vi "poly_recursive_compare_cluster_element(s).vi"(6 "stop after 1st one?":bool, 7 "delimiter (/)":string="/", 8 "error in (no error)":errorcluster, 10 "Data":variant, 11 "Cluster":variant) -> (0 "error out":errorcluster, 1 "field names":string[](array[string]), 2 "found?":bool, 3 "Cluster out":variant)   [LabVIEW 2015]
uses:
  <vilib>/Utility/Data Type/NI_Data Type.lvlib
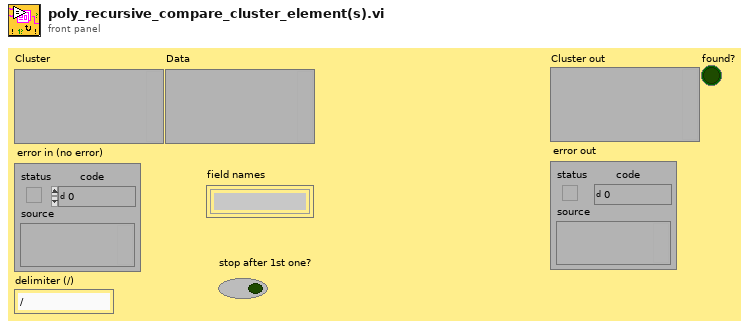
[diagram p1: front panel]
types:
  T1 = typedef "NI_Data Type.lvlib/Data Type.ctl" = enum8{"Invalid Type", "Void", "I8", "I16", "I32", "I64", "U8", "U16", "U32", "U64", "Single Float", "Double Float", "Extended Float", "Single Complex", "Double Complex", "Extended Complex", "Enum U8", "Enum U16", "Enum U32", "Enum U64", "Single Float With Unit", "Double Float With Unit", "Extended Float With Unit", "Single Complex with Unit", "Double Complex with Unit", "Extended Complex with Unit", "Boolean", "String", "Path", "Picture", "Tag", "Array", "Cluster", "Variant", "LV Variant", "Waveform", "Timestamp", "Digital Waveform", "Digital Data", "ExpressData", "Refnum", "External Data", "VI", "Poly VI", "LabVIEW Class Instance", "Fixed Point"}
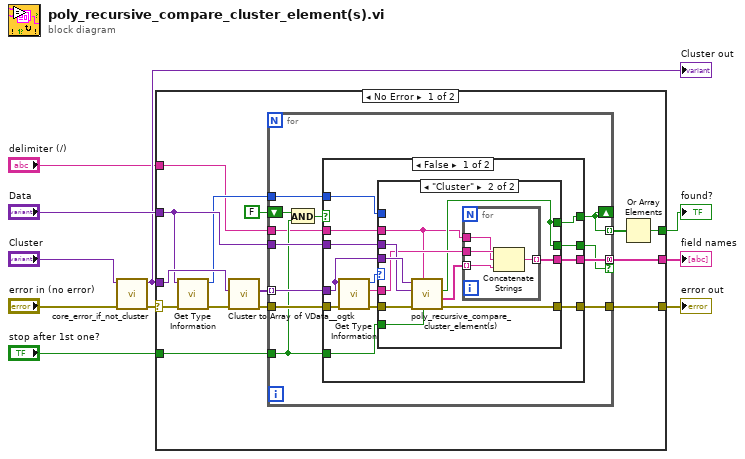
[diagram p0: block diagram]
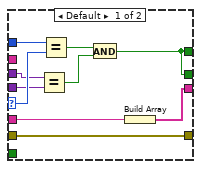
[diagram p2: hidden frame]
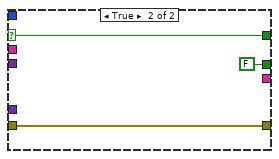
[diagram p3: hidden frame]
diagram:
  n1 = call "core_error_if_not_cluster.vi"("Error in"="error in (no error)", "Cluster"="Cluster") -> ("Error out"=w2:errorcluster, "Cluster duplicate"=w3:variant)  [unwired: 8 in]
  "Cluster out" <- w3
  n2 = case shown="No Error" w2 {
    selector: w2 -> [w12 w77]
    tunnel: w3 -> [w23 _]
    tunnel: "Data" -> [w20 _]
    tunnel: [w16 w77] -> w9
    tunnel: [w21 _] -> w8
    tunnel: "stop after 1st one?" -> [w14 _]
    tunnel: [w15 _] -> w6
    tunnel: "delimiter (/)" -> [w11 _]
    frame No Error {
      n3 = call <vilib>:"Get Type Information.vi"("error in (no error)"=w12, "Variant"=w20) -> ("error out"=w17:errorcluster, "Type"=w19:T1)  [unwired: 5 in, 3 out]
      n4 = call <userlib>:"Cluster to Array of VData__ogtk.vi"("error in (no error)"=w17, "Cluster"=w23) -> ("error out"=w18:errorcluster, "Array of VData"=w24:variant[])  [unwired: 8 in]
      n5 = for {
        tunnel: w24 -> [w36] mode=indexing
        tunnel: w20 -> [w35]
        tunnel: [w33] -> w16
        tunnel: w18 -> [w34]
        tunnel: [w32] -> w22 mode=indexing
        shift-right: [w32] -> _
        shift-left: FALSE ("found?") -> [w28]
        tunnel: w14 -> [w26]
        tunnel: w19 -> [w31]
        tunnel: [w30] -> w15 mode=concatenating if=w29
        tunnel: w11 -> [w25]
        n6 = And(x=w28, y=w26) -> (x .and. y?=w27:bool)
        n7 = case shown="False" w27 {
          selector: w27 -> [_ w75]
          tunnel: w36 -> [w49 _]
          tunnel: w35 -> [w47 _]
          tunnel: w34 -> [w46 w74]
          tunnel: [w44 w74] -> w33
          tunnel: [w42 w75] -> w32
          tunnel: w31 -> [w41 _]
          tunnel: [w40 _] -> w30
          tunnel: [w39 FALSE] -> w29
          tunnel: w26 -> [w38 _]
          tunnel: w25 -> [w37 _]
          frame False {
            n8 = call <vilib>:"Get Type Information.vi"("error in (no error)"=w46, "Variant"=w49) -> ("error out"=w45:errorcluster, "Name"=w43:string, "Type"=w48:T1)  [unwired: 5 in, 2 out]
            n9 = case shown="\"Cluster\"" w48 {
              selector: w48 -> [w58 _]
              tunnel: w49 -> [w56 w69]
              tunnel: w47 -> [w57 w68]
              tunnel: w45 -> [w52 w67]
              tunnel: [w52 w63] -> w44
              tunnel: w43 -> [w55 w65]
              tunnel: [w53 w62] -> w42
              tunnel: w41 -> [w59 _]
              tunnel: [w54 w64] -> w40
              tunnel: [w53 w62] -> w39
              tunnel: w38 -> [_ w61]
              tunnel: w37 -> [_ w60]
              frame Default {
                n10 = Equal?(x=w57, y=w56) -> (x = y?=w50:bool)
                n11 = Equal?(x=w59, y=w58) -> (x = y?=w51:bool)
                n12 = And(x=w51, y=w50) -> (x .and. y?=w53:bool)
                n13 = Build Array(w55) -> (w54:string[])
              }
              frame "Cluster" {
                n14 = call "poly_recursive_compare_cluster_element(s).vi"("stop after 1st one?"=w61, "delimiter (/)"=w60, "error in (no error)"=w67, "Data"=w68, "Cluster"=w69) -> ("error out"=w63:errorcluster, "field names"=w66:string[], "found?"=w62:bool)  [unwired: 3 in, 1 out]
                n15 = for {
                  tunnel: w66 -> [w72] mode=indexing
                  tunnel: w65 -> [w73]
                  tunnel: [w71] -> w64 mode=indexing
                  tunnel: w60 -> [w70]
                  n16 = Concatenate Strings(w73, w70, w72) -> (w71:string)
                }
              }
            }
          }
          frame True {
          }
        }
      }
      n17 = Or Array Elements(Boolean array=w22) -> (logical OR=w21:bool)
    }
    frame Error {
    }
  }
  "error out" <- w9
  "found?" <- w8
  "field names" <- w6
